vi "test_LoadCommandlineArgs_InvalidParameter.vi"() -> (3 "Pass?":bool)   [LabVIEW 2019, in "Tests.SolutionBuilder.lvlib"]
uses:
  Tests.SolutionBuilder.lvlib
  SolutionBuilder/Community/Options.ctl
  SolutionBuilder/SolutionBuilder.lvclass
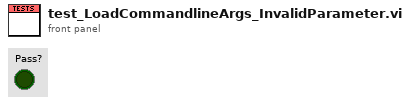
[diagram p1: front panel]
types:
  T1 = typedef "SolutionBuilder.lvlib/SolutionBuilder.lvclass/Options.ctl" = cluster{"Path":path, "Preview?":bool, "Quiet?":bool, "Log file":path, "Success file":path, "Rebuild?":bool, "Keep split projects?":bool, "Version string":string}
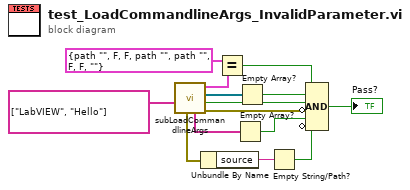
[diagram p0: block diagram]
diagram:
  n1 = call "subLoadCommandlineArgs.vi"("App.Args"=string[] ["LabVIEW", "Hello"]) -> ("error out"=w6:errorcluster, "From command line?"=w12:bool, "Pre-built libraries"=w9:refnum<class "ProjectItem.lvclass">[], "Options"=w8:T1, "Active targets"=w4:string[], "warnings out"=w3:errorcluster)  [unwired: 5 in]
  n2 = Unbundle By Name(w3) -> ("source"=w5:string)
  n3 = Equal?(x=T1 {"Path"=path "", "Preview?"=FALSE, "Quiet?"=FALSE, "Log file"=path "", "Success file"=path "", "Rebuild?"=FALSE, "Keep split projects?"=FALSE, "Version string"=""} ("Options"), y=w8) -> (x = y?=w11:bool)
  n4 = Empty Array?(array=w4) -> (empty?=w2:bool)
  n5 = Empty Array?(array=w9) -> (empty?=w10:bool)
  n6 = Empty String/Path?(string/path=w5) -> (empty?=w1:bool)
  n7 = Compound Arithmetic op=AND(w11, w10, w12, invert w6, w2, invert w1) -> (→"Pass?":bool)
